vi "RandomNumberChart.vi"() -> ()   [LabVIEW 2019]
panel:
  in  "stop":bool
  out "Waveform Chart":dbl(graph)
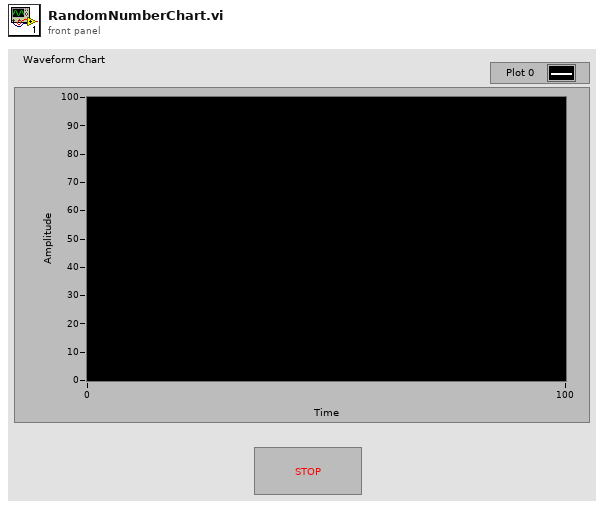
[diagram p1: front panel]
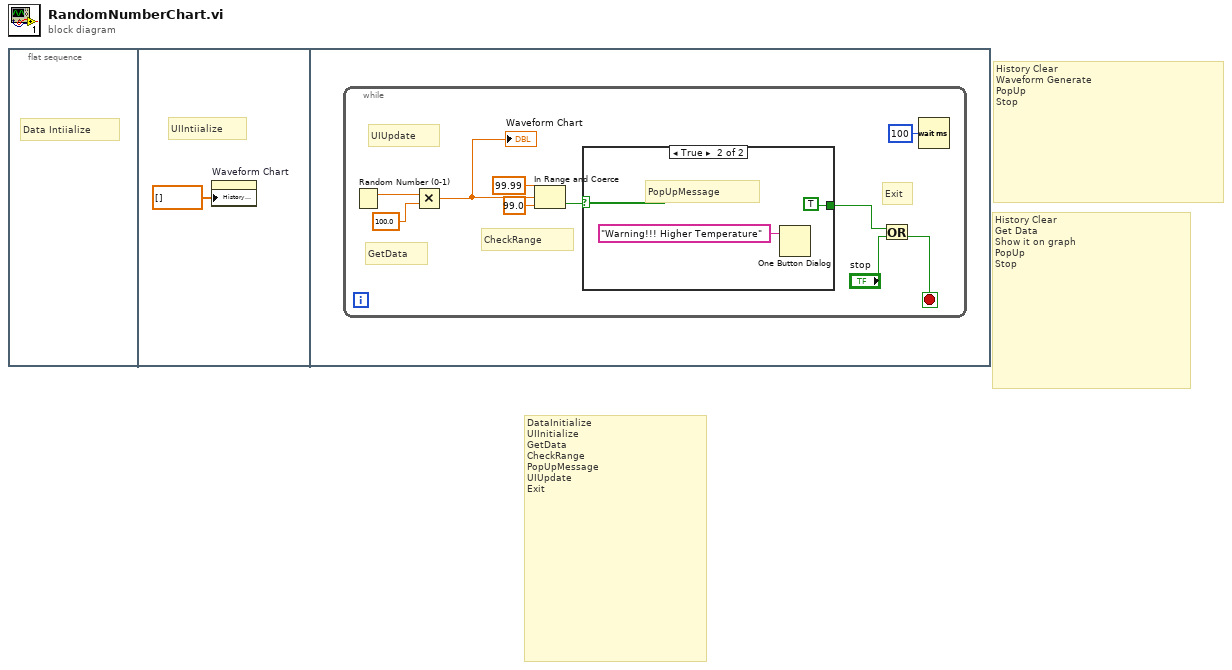
[diagram p0: block diagram]
diagram:
  # "DataInitialize\nUIInitialize\nGetData\nCheckRange\nPopUpMessage\nUIUpdate\nExit"
  # "History Clear\nGet Data\nShow it on graph\nPopUp\nStop"
  # "History Clear\nWaveform Generate\nPopUp\nStop"
  n1 = flat-sequence {
    frame #0 {
      # "Data Intiialize"
    }
    frame #1 {
      # "UIIntiialize"
      n2 = property on="Waveform Chart" class="WFChart (strict)"("History Data"=dbl[] []) -> ()  [unwired: 2 in, 2 out]
    }
    frame #2 {
      n3 = while {
        stop <- w4 stop-if-true
        # "Exit"
        # "UIUpdate"
        # "CheckRange"
        # "GetData"
        n4 = Random Number (0-1)() -> (number: 0 to 1=w11:dbl)
        n5 = Multiply(x=w11, y=100.0) -> (x*y=w2:dbl)
        "Waveform Chart" <- w2
        n6 = In Range and Coerce(upper limit=99.99, x=w2, lower limit=99.0) -> (In Range?=w5:bool)  [unwired: 1 out]
        n7 = case shown="True" w5 {
          tunnel: [_ TRUE] -> w3
          frame False {
          }
          frame True {
            # "PopUpMessage"
            n8 = One Button Dialog(message="Warning!!! Higher Temperature") -> ()  [unwired: 1 in, 1 out]
          }
        }
        n9 = Or(x=w3, y="stop") -> (x .or. y?=w4:bool)
        n10 = Wait (ms)(milliseconds to wait=u32 100) -> ()  [unwired: 1 out]
      }
    }
  }
